vi "SEA_9811_Word_to_EU_Array.vi"(7 "Channel":u32, 8 "error in (no error)":errorcluster, 10 "ARINC word in":T1 {"ARINC word" format="%032b"}, 11 "SEA9811_RT_data in":T3 {"Tx"."Tx Refs (Data,Trig)"."Data Reference" format="%.0x"}) -> (0 "error out":errorcluster, 3 "SEA9811_RT_data out":T3 {"Tx"."Tx Refs (Data,Trig)"."Data Reference" format="%.0x"})   [LabVIEW 2012]
doc: "puts received ARINC word and timestamp into correct positions in DBL array.\n\nFor no only for channel 0"
uses:
  Typdefs/SEA9811_RT_data_cluster.ctl
  <userlib>/_FPGA Interface Advanced Tools/FPGA Interface Base/FPGA Interface Base.lvclass
  Typdefs/FPGA ref.ctl
  Typdefs/channel.ctl
  Typdefs/received word.ctl
  Typdefs/SEA9811_FPGA_FP_Addresses.ctl
  <vilib>/NI Veristand/Custom Device API/Block Data Reference.ctl
  <vilib>/NI Veristand/Custom Device API/Data Reference.ctl
  Typdefs/ARINC word cluster.ctl
  Typdefs/ARINC word.ctl
  <vilib>/NI Veristand/Custom Device API/Custom Device API.lvlib
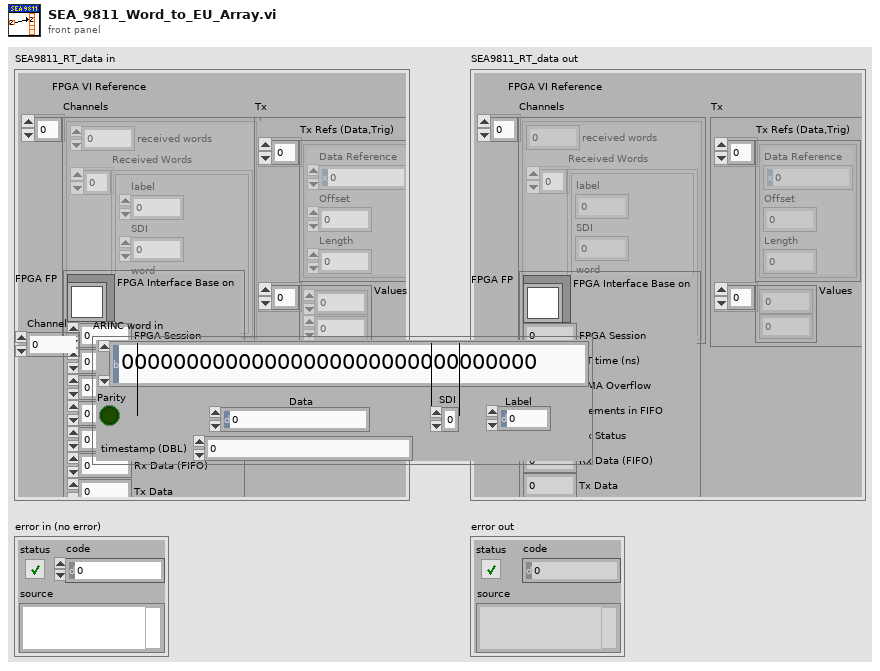
[diagram p1: front panel]
types:
  T1 = typedef "ARINC word cluster.ctl" = cluster{"ARINC word":T2, "Label":u8, "SDI":u8, "Data":u32, "Parity":bool, "timestamp (DBL)":dbl}
  T2 = typedef "ARINC word.ctl" = u32
  T3 = typedef "SEA9811_RT_data_cluster.ctl" = cluster{"FPGA VI Reference":T4, "Channels":T5[], "FPGA FP":T7, "Tx":cluster{"Tx Refs (Data,Trig)":T8[], "Values":dbl[]}}
  T4 = typedef "FPGA ref.ctl" = refnum<k20>
  T5 = typedef "channel.ctl" = cluster{"received words":u32, "Received Words":T6[]}
  T6 = typedef "received word.ctl" = cluster{"label":u8, "SDI":u8, "word":u32, "timestamp":dbl}
  T7 = typedef "SEA9811_FPGA_FP_Addresses.ctl" = cluster{"FPGA Interface Base on":refnum<class "FPGA Interface Base.lvclass">, "FPGA Session":u32, "RT time (ns)":u32, "DMA Overflow":u32, "Elements in FIFO":u32, "Rx Status":u32, "Rx Data (FIFO)":u32, "Tx Data":u32, "Transmit Data":u32}
  T8 = typedef "Custom Device API.lvlib/Block Data Reference.ctl" = cluster{"Data Reference":T9, "Offset":i32, "Length":i32}
  T9 = typedef "Custom Device API.lvlib/Data Reference.ctl" = i32
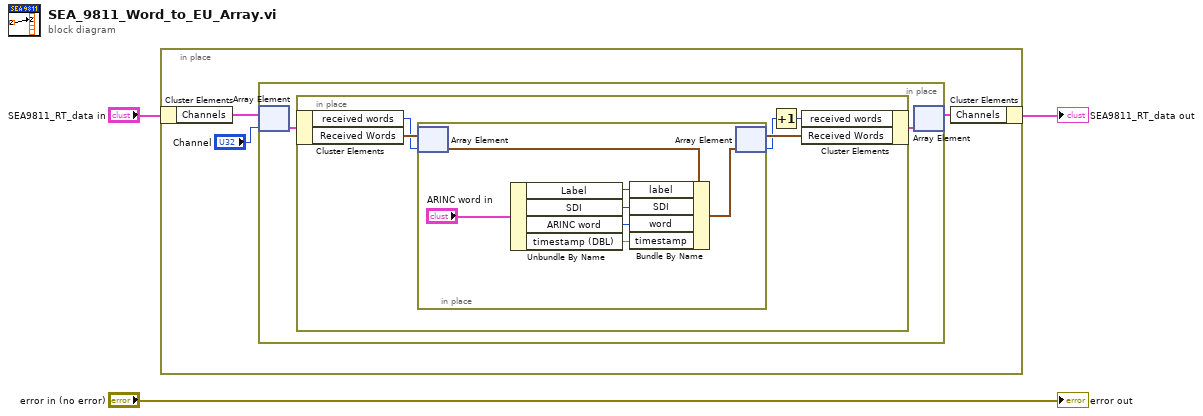
[diagram p0: block diagram]
diagram:
  n1 = in-place {
    n2 = in-place-cluster #1("SEA9811_RT_data in") -> ("Channels"=w6:T5[])
    n3 = in-place {
      n4 = in-place-array #2(w6, "Channel") -> (w8:T5)
      n5 = in-place {
        n6 = in-place-cluster #3(w8) -> ("received words"=w12:u32, "Received Words"=w13:T6[])
        n7 = in-place {
          n8 = in-place-array #4(w13, w12) -> (w18:T6)
          n9 = Unbundle By Name("ARINC word in") -> ("Label"=w19:u8, "SDI"=w17:u8, "ARINC word"=w16:T2, "timestamp (DBL)"=w15:dbl)
          n10 = Bundle By Name(cluster=w18, "label"=w19, "SDI"=w17, "word"=w16, "timestamp"=w15) -> (w14:T6)
          n11 = in-place-array #4(w14) -> (w10:T6[], w9:i32)
        }
        n12 = Increment(x=w9) -> (x+1=w11:i32)
        n13 = in-place-cluster #3("received words"=w11, "Received Words"=w10) -> (w7:T5)
      }
      n14 = in-place-array #2(w7) -> (w4:T5[])  [unwired: 1 out]
    }
    n15 = in-place-cluster #1("Channels"=w4) -> (→"SEA9811_RT_data out":T3)
  }
  "error out" <- "error in (no error)"
